vi "test-SetGetControlValue.vi"() -> (0 "errors":errorcluster[](array[cluster]))   [LabVIEW 2021]
uses:
  <vilib>/regexp/Match Regular Expression.xnode
panel:
  out "Variant":variant=variant(dbl 1.0)
  in  "Tab Control":enum32{"Page 1", "Page 2"}(tab)
  in  "Multiline\nwith\tTAB":string
  in  "NumericInPanel":dbl
  in  "Tab Control 2":enum32{"Page 1", "Page 2"}(tab)
  in  "StringInPanel":string
  in  "StringInPanel2":string
  in  "NumericInPanel2":dbl
  out "StringInd":string
  out "NumericInd":dbl
  in  "ClusterArray":cluster{"DBL":dbl, "U16":u16, "String":string}[](array[cluster])=[{"DBL"=2.0, "U16"=3, "String"="abc"}, {"DBL"=0.0, "U16"=0, "String"="aaa"}]
  in  "Cluster":T1={"DBL"=1.2, "U16"=3, "String"="bcd", "Ring U16"=3, "Ring EXT"=1.0, "Array"=[1.0, -1.0], "Boo/lean[2]"=FALSE} {"Ring EXT" items=["one", "three"]; "Ring U16" items=["one"=1, "three"=3]}
  in  "Array I32 2D":i32[][](array[numeric])=[[0, -1, 2], [3, 4, 5]]
  in  "Array I32":i32[](array[numeric])=[-1, 1, 2]
  in  "Enum":enum16{"zero", "one", "two"}(ring)
  in  "Ring 2":ext(ring)=3.3 items=["one", "three"]
  in  "Ring":u16(ring)=4 items=["one"=1, "three"=3]
  in  "Path":path
  in  "Combo Box 2":string(combo)="item1"
  in  "Combo Box":string(combo)="value1"
  in  "String":string="a\tb\nc\""
  in  "Radio Buttons":enum32{"Radio1", "Radio2"}(radio)
  in  "Boolean":bool
  in  "Color Box":u32(colorbox)
  in  "Scrollbar":dbl(c297)
  in  "Knob":dbl(knob) scale=0.0..10.0
  in  "Slide":dbl(slide) scale=0.0..10.0
  in  "Numeric U8":u8
  in  "Numeric CXT":cxt=10.0-0.30000000000000000001i
  in  "Numeric EXT":dbl=100.0
  out "Result":string="# Radio Buttons\nRadio Buttons=\"Radio2\"; Radio Buttons==\"Radio2\";\nRadio Buttons=0; Radio Buttons==\"Radio1\";"
  out "error":bool
  in  "CommandArray":T2(array[cluster])=[{"command"="# Numeric EXT 読み書きできるか\nNumeric EXT=3; Numeric EXT==3 # 一旦 3 にして\nNumeric EXT=0; Numeric EXT==0 # 0 に戻す", "result"="", "error"=FALSE}, {"command"="# Numeric EXT いろんな書き方\nNumeric EXT=1.0;Numeric EXT==1; # %f\nNumeric EXT=1E1;Numeric EXT==10; # %e\nNumeric EXT=\"1E2\";Numeric EXT==100; # 文字列でもOK", "result"="", "error"=FALSE}, {"command"="# 複素数\nNumeric CXT=1; Numeric CXT==\"1 +0 i\"\nNumeric CXT=-1; Numeric CXT==\"-1 +0 i\"\nNumeric CXT=\"0 +3.2 i\"; Numeric CXT==\"0 +3.2 i\"\nNumeric CXT=\"0 + i\"; Numeric CXT==\"0 +1 i\"\nNumeric CXT=\"0 - i\"; Numeric CXT==\"0 -1 i\"\nNumeric CXT=\"0 - 3.2 i\"; Numeric CXT==\"0 -3.2 i\"\nNumeric CXT=\"1e1 - 3e-1 i\"; Numeric CXT==\"10 -0.3 i\"", "result"="", "error"=FALSE}, {"command"="# Unsigned 8 bits\nNumeric U8=3; Numeric U8==3;\nNumeric U8=256; Numeric U8==255; # オーバーフローは飽和する\nNumeric U8=-2; Numeric U8==0; # アンダーフローも飽和する", "result"="", "error"=FALSE}, {"command"="# スライダー・Knob\nSlide=6; Slide==6; Slide=0; Slide==0; \nKnob=2; Knob==2; Knob=0; Knob==0", "result"="", "error"=FALSE}, {"command"="# Scrollbar\nScrollbar=10; Scrollbar==10;\nScrollbar=0.1; Scrollbar==0.1;\nScrollbar=0; Scrollbar==0;", "result"="", "error"=FALSE}, {"command"="# ColorBox\nColor Box=10000;Color Box==10000;\nColor Box=0;Color Box==0;", "result"="", "error"=FALSE}, {"command"="# Boolean\nBoolean=true; Boolean=false;\nBoolean=1; Boolean=0 # 数値でもいい", "result"="", "error"=FALSE}, {"command"="# Radio Buttons\nRadio Buttons=\"Radio2\"; Radio Buttons==\"Radio2\";\nRadio Buttons=0; Radio Buttons==\"Radio1\";", "result"="", "error"=FALSE}, {"command"="# String\nString=\"abc\"; String==\"abc\"; \nString=def; String==\"def\";  # これは許される\n# String=true; String==\"true\";  # これはエラーになる\n# String=0; String==\"0\";  # これらはエラーになる\nString=\"\"; String==\"\"; \nString=\"a\\tb\\nc\\\"\"; String==\"a\\tb\\nc\\\"\"; # エスケープシーケンス ", "result"="", "error"=FALSE}, {"command"="# Combo Box\nCombo Box=\"item1\"; Combo Box==\"item1\"; \nCombo Box=\"value1\"; Combo Box==\"value1\"; # 表示は item1 になる ", "result"="", "error"=FALSE}, {"command"="# Combo Box (Force Defined Value)\nCombo Box 2=\"item2\"; Combo Box 2==\"item2\"; \nCombo Box 2=\"\"; Combo Box 2==\"\"; \nCombo Box 2=\"value1\"; Combo Box 2==\"value1\"; # 表示は item1 になる\nCombo Box 2=\"undefined\"; Combo Box 2==\"undefined\"; # 代入する分には入れられる \nCombo Box 2=\"item1\"; Combo Box 2==\"item1\"; ", "result"="", "error"=FALSE}, {"command"="# Path\nPath=\"C:\\\\\"; Path==\"C:\\\\\"; \nPath=\"\"; Path==\"\"; ", "result"="", "error"=FALSE}, {"command"="# Ring\nRing=\"three\"; Ring==\"three\"; \nRing=\"one\"; Ring==\"one\"; \nRing=3; Ring==\"three\";  # 数値でも指定可能\nRing=0; Ring==\"<0>\"; # 範囲外の値も読み書きできる\nRing=\"<4>\"; Ring==\"<4>\"; # 文字列でもOK", "result"="", "error"=FALSE}, {"command"="# Ring メニュー（形は違うが機能は同じ？\nRing 2=\"three\"; Ring 2==\"three\"; \nRing 2=\"one\"; Ring 2==\"one\"; \nRing 2=3; Ring 2==\"three\";  # 数値でも指定可能\nRing 2=\"<3.2>\"; Ring 2==\"<3.2>\"\nRing 2=3.3; Ring 2==\"<3.3>\"", "result"="", "error"=FALSE}, {"command"="# Enum\nEnum=1; Enum==\"one\"\nEnum=\"two\"; Enum==\"two\"\nEnum=0; Enum==\"zero\"\nEnum=3; Enum==\"two\" # 範囲外の値は飽和する\nEnum=-1; Enum==\"zero\" # 範囲外の値は飽和する", "result"="", "error"=FALSE}, {"command"="# Array I32\nArray I32=[]; Array I32==[]\nArray I32=[0,1,2]; Array I32==[0,1,2]\nArray I32[0]=-1; Array I32==[-1,1,2]\n# Array I32[3]=-1; Array I32[-1]=-1 # Array index out of range エラーが出る", "result"="", "error"=FALSE}, {"command"="# Array I32 2D 多次元配列も可能\nArray I32 2D=[[0,0],[]]; Array I32 2D==[[0,0],[]]\nArray I32 2D=[[2,3],[0,1,2,3,4,5]];Array I32 2D==[[2,3],[0,1,2,3,4,5]]\nArray I32 2D[0,1]=-1;Array I32 2D==[[2,3],[0,-1,2,3,4,5]]\n# Array I32 2D[2,1]=-1; # Array index out of range.", "result"="", "error"=FALSE}, {"command"="# Cluster\nCluster={\"DBL\":0.1,\"U16\":3,\"String\":\"a\",\"Ring U16\":1, \"Ring EXT\":1,\"Array\":[]}\nCluster=={\"DBL\":0.1,\"U16\":3,\"String\":\"a\",\"Ring U16\":\"one\",\"Ring EXT\":\"one\",\"Array\":[]}\nCluster={0:0.2,3:\"three\"} # メンバー番号でもアクセスできる 一部のメンバーだけ指定してもいい\nCluster=={\"DBL\":0.2,\"U16\":3,\"String\":\"a\",\"Ring U16\":\"three\",\"Ring EXT\":\"one\",\"Array\":[]}\nCluster/DBL=1.2 # / でパスを指定して１つのメンバーだけにアクセスすることもできる\nCluster=={\"DBL\":1.2,\"U16\":3,\"String\":\"a\",\"Ring U16\":\"three\",\"Ring EXT\":\"one\",\"Array\":[]}\nCluster/DBL==1.2\nCluster/String=\"bcd\"\nCluster/String==\"bcd\"\nCluster/Array=[1,2]\nCluster/Array[1]=-1\nCluster/Array==[1,-1]", "result"="", "error"=FALSE}, {"command"="# ClusterArray\nClusterArray=[{DBL:2,U16:3,String:\"abc\"},{DBL:0,U16:-1,String:\"def\"}] # U16 に -1 は入らない\nClusterArray==[{\"DBL\":2,\"U16\":3,\"String\":\"abc\"},{\"DBL\":0,\"U16\":0,\"String\":\"def\"}]\nClusterArray[1]/DBL==0\nClusterArray[1]/String=\"aaa\"\nClusterArray[1]/String==\"aaa\"", "result"="", "error"=FALSE}, {"command"="# 表示器も扱える\nNumericInd=2; NumericInd==2\nNumericInd=0; NumericInd==0\nStringInd=\"aa\"; StringInd==\"aa\"\nStringInd=\"\"; StringInd==\"\"", "result"="", "error"=FALSE}, {"command"="# ページコントロールの各ページは平坦化される\nNumericInPanel=2; NumericInPanel==2; NumericInPanel=0; NumericInPanel==0\nNumericInPanel2=2; NumericInPanel2==2; NumericInPanel2=0; NumericInPanel2==0\nStringInPanel=\"aa\"; StringInPanel==\"aa\"; StringInPanel=\"\"; StringInPanel==\"\"\nStringInPanel2=\"aa\"; StringInPanel2==\"aa\"; StringInPanel2=\"\"; StringInPanel2==\"\"", "result"="", "error"=FALSE}, {"command"="# Sub Panel は一段下がる\nSub Panel/Numeric=1; Sub Panel/Numeric==1; Sub Panel/Numeric=0; Sub Panel/Numeric==0", "result"="", "error"=FALSE}, {"command"="# Variant 部分的なサポートしかない\n# 文字列、Boolean はOK。数値は部分的サポート。他は無理。\nVariant=\"abc\"; Variant==\"abc\"\nVariant=true; Variant==true\nVariant=false; Variant==false\n# 実数値も読み書きできるが書き込み時は常に EXT 型になる\nVariant=1.0; Variant==1", "result"="", "error"=FALSE}] caption="[テストスクリプト＆実行結果]\nテストスクリプトをここで一時的に変更して左上のボタンで再実行できるが\n内容は保存されないため必要ならダイアグラムのスクリプト欄を変更すること。"
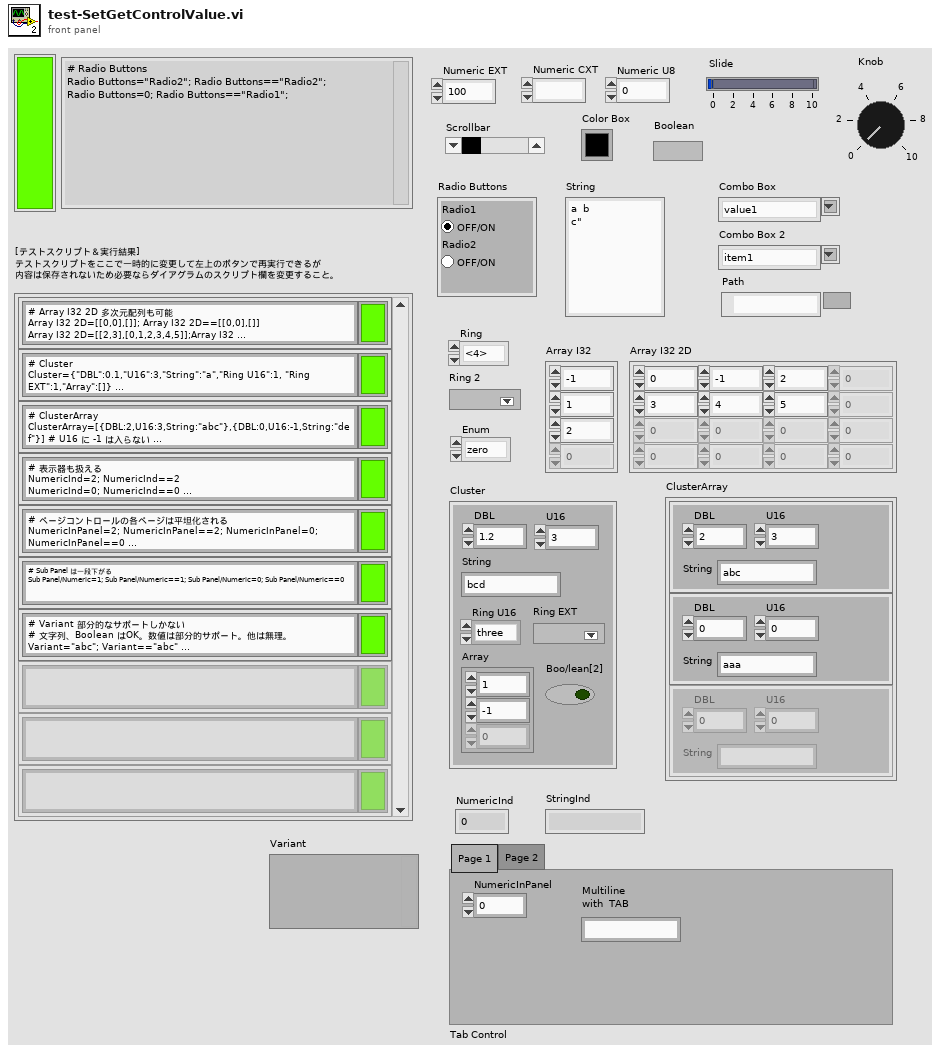
[diagram p1: front panel]
types:
  T1 = cluster{"DBL":dbl, "U16":u16, "String":string, "Ring U16":u16, "Ring EXT":ext, "Array":dbl[], "Boo/lean[2]":bool}
  T2 = cluster{"command":string, "result":string, "error":bool}[]
  T3 = cluster{"command":string, "result":string, "error":bool}
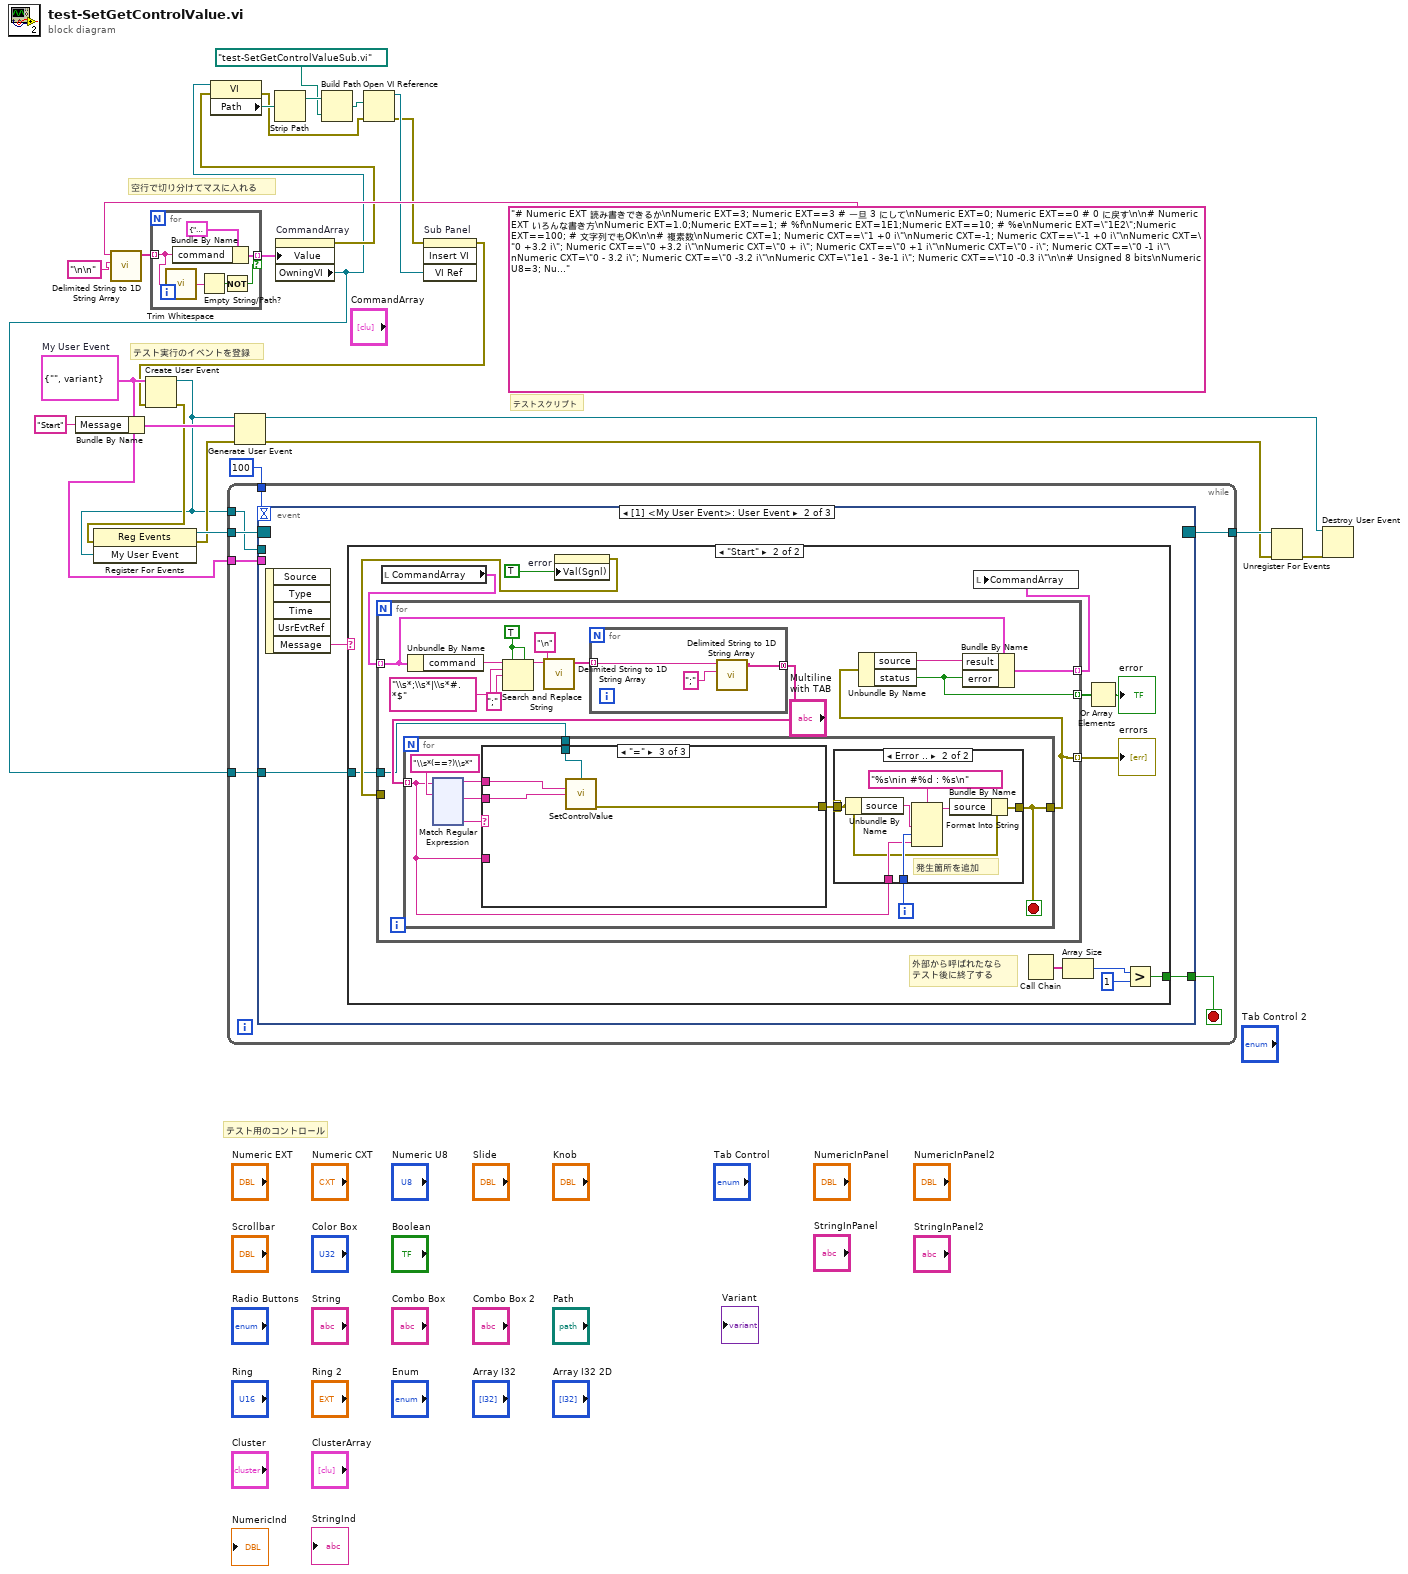
[diagram p0: block diagram]
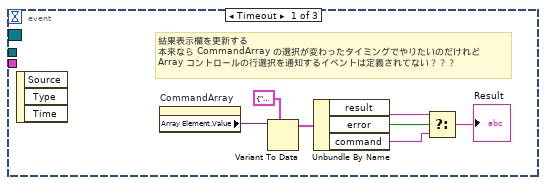
[diagram p2: hidden frame]
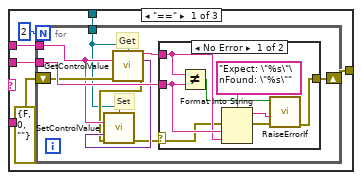
[diagram p5: hidden frame]
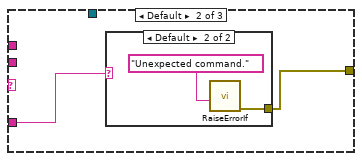
[diagram p7: hidden frame]
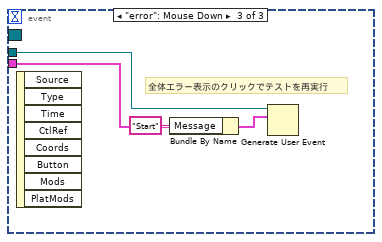
[diagram p9: hidden frame]
diagram:
  w16 = cluster{"Message":string, "Parameter":variant} {"Message"="", "Parameter"=variant}  # My User Event
  # "テスト用のコントロール"
  # "テスト実行のイベントを登録"
  # "空行で切り分けてマスに入れる"
  # "テストスクリプト"
  n1 = Bundle By Name(cluster=w16, "Message"="Start") -> (w19:cluster{"Message":string, "Parameter":variant})
  n2 = call <vilib>:"Delimited String to 1D String Array.vi"("delimiter"="\n\n", "delimited string"="# Numeric EXT 読み書きできるか\nNumeric EXT=3; Numeric EXT==3 # 一旦 3 にして\nNumeric EXT=0; Numeric EXT==0 # 0 に戻す\n\n# Numeric EXT いろんな書き方\nNumeric EXT=1.0;Numeric EXT==1; # %f\nNumeric EXT=1E1;Numeric EXT==10; # %e\nNumeric EXT=\"1E2\";Numeric EXT==100; # 文字列でもOK\n\n# 複素数\nNumeric CXT=1; Numeric CXT==\"1 +0 i\"\nNumeric CXT=-1; Numeric CXT==\"-1 +0 i\"\nNumeric CXT=\"0 +3.2 i\"; Numeric CXT==\"0 +3.2 i\"\nNumeric CXT=\"0 + i\"; Numeric CXT==\"0 +1 i\"\nNumeric CXT=\"0 - i\"; Numeric CXT==\"0 -1 i\"\nNumeric CXT=\"0 - 3.2 i\"; Numeric CXT==\"0 -3.2 i\"\nNumeric CXT=\"1e1 - 3e-1 i\"; Numeric CXT==\"10 -0.3 i\"\n\n# Unsigned 8 bits\nNumeric U8=3; Numeric U8==3;\nNumeric U8=256; Numeric U8==255; # オーバーフローは飽和する\nNumeric U8=-2; Numeric U8==0; # アンダーフローも飽和する\n\n# スライダー・Knob\nSlide=6; Slide==6; Slide=0; Slide==0; \nKnob=2; Knob==2; Knob=0; Knob==0\n\n# Scrollbar\nScrollbar=10; Scrollbar==10;\nScrollbar=0.1; Scrollbar==0.1;\nScrollbar=0; Scrollbar==0;\n\n# ColorBox\nColor Box=10000;Color Box==10000;\nColor Box=0;Color Box==0;\n\n# Boolean\nBoolean=true; Boolean=false;\nBoolean=1; Boolean=0 # 数値でもいい\n\n# Radio Buttons\nRadio Buttons=\"Radio2\"; Radio Buttons==\"Radio2\";\nRadio Buttons=0; Radio Buttons==\"Radio1\";\n\n# String\nString=\"abc\"; String==\"abc\"; \nString=def; String==\"def\";  # これは許される\n# String=true; String==\"true\";  # これはエラーになる\n# String=0; String==\"0\";  # これらはエラーになる\nString=\"\"; String==\"\"; \nString=\"a\\tb\\nc\\\"\"; String==\"a\\tb\\nc\\\"\"; # エスケープシーケンス \n\n# Combo Box\nCombo Box=\"item1\"; Combo Box==\"item1\"; \nCombo Box=\"value1\"; Combo Box==\"value1\"; # 表示は item1 になる \n\n# Combo Box (Force Defined Value)\nCombo Box 2=\"item2\"; Combo Box 2==\"item2\"; \nCombo Box 2=\"\"; Combo Box 2==\"\"; \nCombo Box 2=\"value1\"; Combo Box 2==\"value1\"; # 表示は item1 になる\nCombo Box 2=\"undefined\"; Combo Box 2==\"undefined\"; # 代入する分には入れられる \nCombo Box 2=\"item1\"; Combo Box 2==\"item1\"; \n\n# Path\nPath=\"C:\\\\\"; Path==\"C:\\\\\"; \nPath=\"\"; Path==\"\"; \n\n# Ring\nRing=\"three\"; Ring==\"three\"; \nRing=\"one\"; Ring==\"one\"; \nRing=3; Ring==\"three\";  # 数値でも指定可能\nRing=0; Ring==\"<0>\"; # 範囲外の値も読み書きできる\nRing=\"<4>\"; Ring==\"<4>\"; # 文字列でもOK\n\n# Ring メニュー（形は違うが機能は同じ？\nRing 2=\"three\"; Ring 2==\"three\"; \nRing 2=\"one\"; Ring 2==\"one\"; \nRing 2=3; Ring 2==\"three\";  # 数値でも指定可能\nRing 2=\"<3.2>\"; Ring 2==\"<3.2>\"\nRing 2=3.3; Ring 2==\"<3.3>\"\n\n# Enum\nEnum=1; Enum==\"one\"\nEnum=\"two\"; Enum==\"two\"\nEnum=0; Enum==\"zero\"\nEnum=3; Enum==\"two\" # 範囲外の値は飽和する\nEnum=-1; Enum==\"zero\" # 範囲外の値は飽和する\n\n# Array I32\nArray I32=[]; Array I32==[]\nArray I32=[0,1,2]; Array I32==[0,1,2]\nArray I32[0]=-1; Array I32==[-1,1,2]\n# Array I32[3]=-1; Array I32[-1]=-1 # Array index out of range エラーが出る\n\n# Array I32 2D 多次元配列も可能\nArray I32 2D=[[0,0],[]]; Array I32 2D==[[0,0],[]]\nArray I32 2D=[[2,3],[0,1,2,3,4,5]];Array I32 2D==[[2,3],[0,1,2,3,4,5]]\nArray I32 2D[0,1]=-1;Array I32 2D==[[2,3],[0,-1,2,3,4,5]]\n# Array I32 2D[2,1]=-1; # Array index out of range.\n\n# Cluster\nCluster={\"DBL\":0.1,\"U16\":3,\"String\":\"a\",\"Ring U16\":1, \"Ring EXT\":1,\"Array\":[],\"Boo/lean[2]\":false}\nCluster=={\"DBL\":0.1,\"U16\":3,\"String\":\"a\",\"Ring U16\":\"one\",\"Ring EXT\":\"one\",\"Array\":[],\"Boo/lean[2]\":false}\nCluster={0:0.2,3:\"three\",\"Boo/lean[2]\":true} # メンバー番号でもアクセスできる 一部のメンバーだけ指定してもいい\nCluster=={\"DBL\":0.2,\"U16\":3,\"String\":\"a\",\"Ring U16\":\"three\",\"Ring EXT\":\"one\",\"Array\":[],\"Boo/lean[2]\":true}\nCluster/DBL=1.2 # / でパスを指定して１つのメンバーだけにアクセスすることもできる\nCluster=={\"DBL\":1.2,\"U16\":3,\"String\":\"a\",\"Ring U16\":\"three\",\"Ring EXT\":\"one\",\"Array\":[],\"Boo/lean[2]\":true}\nCluster/DBL==1.2\nCluster/String=\"bcd\"\nCluster/String==\"bcd\"\nCluster/Array=[1,2]\nCluster/Array[1]=-1\nCluster/Array==[1,-1]\nCluster/Boo\\/lean\\[2]=false # / [ を含むコントロール名をパスで指定する際には \\ でエスケープする\nCluster/Boo\\/lean\\[2]==false\n\n# ClusterArray\nClusterArray=[{DBL:2,U16:3,String:\"abc\"},{DBL:0,U16:-1,String:\"def\"}] # U16 に -1 は入らない\nClusterArray==[{\"DBL\":2,\"U16\":3,\"String\":\"abc\"},{\"DBL\":0,\"U16\":0,\"String\":\"def\"}]\nClusterArray[1]/DBL==0\nClusterArray[1]/String=\"aaa\"\nClusterArray[1]/String==\"aaa\"\n\n# 表示器も扱える\nNumericInd=2; NumericInd==2\nNumericInd=0; NumericInd==0\nStringInd=\"aa\"; StringInd==\"aa\"\nStringInd=\"\"; StringInd==\"\"\n\n# ページコントロールの各ページは平坦化される\nNumericInPanel=2; NumericInPanel==2; NumericInPanel=0; NumericInPanel==0\nNumericInPanel2=2; NumericInPanel2==2; NumericInPanel2=0; NumericInPanel2==0\nStringInPanel=\"aa\"; StringInPanel==\"aa\"; StringInPanel=\"\"; StringInPanel==\"\"\nStringInPanel2=\"aa\"; StringInPanel2==\"aa\"; StringInPanel2=\"\"; StringInPanel2==\"\"\n\n# Sub Panel は一段下がる\nSub Panel/Numeric=1; Sub Panel/Numeric==1\nSub Panel/Numeric=0; Sub Panel/Numeric==0\n\n# Variant 部分的なサポートしかない\n# 文字列、Boolean はOK。数値は部分的サポート。他は無理。\nVariant=\"abc\"; Variant==\"abc\"\nVariant=true; Variant==true\nVariant=false; Variant==false\n# 実数値も読み書きできるが書き込み時は常に EXT 型になる\nVariant=1.0; Variant==1\n\n# Tab Control のページを選択できる(数値かページ名)\nTab Control=1; Tab Control==\"Page 2\"\nTab Control=0; Tab Control==\"Page 1\"\nTab Control=\"Page 2\"; Tab Control==\"Page 2\"\n\n# 名前のエスケープ\nMultiline\\nwith\\tTAB=\"\"; Multiline\\nwith\\tTAB==\"\"\nMultiline\\nwith\\tTAB=\"Hello!\"; Multiline\\nwith\\tTAB==\"Hello!\"\n" ("Script")) -> ("string array"=w13:string[])  [unwired: 9 in]
  n3 = for {
    tunnel: w13 -> [w27] mode=indexing
    tunnel: [w32] -> w12 mode=indexing if=w29
    n4 = call <vilib>:"Trim Whitespace.vi"("string"=w27) -> ("trimmed string"=w28:string)  [unwired: 1 in]
    n5 = Bundle By Name(cluster=T3 {"command"="", "result"="", "error"=FALSE} ("Cluster"), "command"=w27) -> (w32:T3)
    n6 = Empty String/Path?(string/path=w28) -> (empty?=w30:bool)
    n7 = Not(x=w30) -> (.not. x?=w29:bool)
  }
  n8 = property on="CommandArray" class="Arr (strict)"("Value"=w12) -> (error out=w4:errorcluster, "OwningVI"=w1:refnum<vi>)  [unwired: 2 in, 1 out]
  n9 = property class="VI"(reference=w1, error in=w4) -> (error out=w3:errorcluster, "Path"=w9:path)  [unwired: 1 out]
  n10 = Strip Path(path=w9) -> (stripped path=w8:path)  [unwired: 1 out]
  n11 = Build Path(base path=w8, name or relative path=path "test-SetGetControlValueSub.vi") -> (appended path=w6:path)
  n12 = Open VI Reference(vi path=w6, error in (no error)=w3) -> (vi reference=w5:refnum<vi>, error out=w2:errorcluster)  [unwired: 4 in]
  n13 = invoke on="Sub Panel" class="SubPnl" method="Insert VI"(error in=w2, "VI Ref"=w5) -> (error out=w10:errorcluster)  [unwired: 2 in, 3 out]
  n14 = Create User Event(user event datatype=w16, error in=w10) -> (user event=w17:refnum<user-event>, error out=w18:errorcluster)
  n15 = register-events(error in=w18, w17) -> (reference out=w26:refnum<event-registration>, error out=w24:errorcluster)  [unwired: 1 in]
  n16 = while {
    tunnel: w26 -> [w39]
    tunnel: [w38] -> w25
    tunnel: w17 -> [w37]
    tunnel: w16 -> [w36]
    tunnel: 100 -> [w35]
    tunnel: w1 -> [w33]
    stop <- w34 stop-if-true
    n17 = event shown="[1] <My User Event>: User Event" {
      selector: w39 -> [_ _ _]
      dyn-events: [_ _ _] -> w38
      timeout: w35 -> [_ _ _]
      tunnel: w37 -> [_ _ w251]
      tunnel: w36 -> [_ _ w249]
      tunnel: [_ w48 _] -> w34
      tunnel: w33 -> [_ w47 _]
      event Timeout {
        # "結果表示欄を更新する\n本来なら CommandArray の選択が変わったタイミングでやりたいのだけれど\nArray コントロールの行選択を通知するイベントは定義されてない？？？"
        n18 = event-data() -> ()  [unwired: 1 in, 3 out]
        n19 = property on="CommandArray" class="Arr (strict)"() -> ("Array Element.Value"=w46:variant)  [unwired: 2 in, 2 out]
        n20 = Variant To Data(type=T3 {"command"="", "result"="", "error"=FALSE} ("Cluster"), Variant=w46) -> (data=w44:T3)  [unwired: 1 in, 1 out]
        n21 = Unbundle By Name(w44) -> ("result"=w42:string, "error"=w43:bool, "command"=w41:string)
        n22 = Select(t=w42, s=w43, f=w41) -> (s? t:f=→"Result":string)
      }
      event User Event {
        n23 = event-data() -> ("Message"=w49:string)  [unwired: 1 in, 4 out]
        n24 = case shown="\"Start\"" w49 {
          tunnel: [_ w53] -> w48
          tunnel: w47 -> [_ w50]
          frame Default {
          }
          frame "Start" {
            # "外部から呼ばれたなら\nテスト後に終了する"
            n25 = local read "CommandArray"() -> (w61:T2)
            n26 = property on="error" class="Bool (strict)"("Val(Sgnl)"=TRUE ("Value (Signaling)")) -> (error out=w51:errorcluster)  [unwired: 2 in, 1 out]
            n27 = for {
              tunnel: w61 -> [w69] mode=indexing
              tunnel: [w67] -> w60 mode=indexing
              tunnel: [w66] -> w59 mode=indexing
              tunnel: [w63] -> w57 mode=indexing
              tunnel: w51 -> [_]
              tunnel: w50 -> [w62]
              w64 = TRUE ("replace all? (F)")
              n28 = Unbundle By Name(w69) -> ("command"=w72:string)
              n29 = Search and Replace String(replace all?=w64, multiline?=w64, input string=w72, search string="\\s*;\\s*|\\s*#.*$", replace string=";" ("replace string (\"\")")) -> (result string=w65:string)  [unwired: 3 in, 3 out]
              n30 = call <vilib>:"Delimited String to 1D String Array.vi"("delimiter"="\n", "delimited string"=w65) -> ("string array"=w74:string[])  [unwired: 9 in]
              n31 = for {
                tunnel: w74 -> [w245] mode=indexing
                tunnel: [w247] -> w70 mode=concatenating
                n32 = call <vilib>:"Delimited String to 1D String Array.vi"("delimiter"=";", "delimited string"=w245) -> ("string array"=w247:string[])  [unwired: 9 in]
              }
              n33 = for {
                tunnel: w70 -> [w77] mode=indexing
                tunnel: [w79] -> w63
                tunnel: w62 -> [w76]
                i -> [w80]
                stop <- w79 stop-if-true
                n34 = xnode "Match Regular Expression"("input string"=w77, "regular expression"="\\s*(==?)\\s*") -> ("before match"=w83:string, "after match"=w82:string, "submatch 1"=w78:string)  [unwired: 4 in, 3 out]
                n35 = case shown="\"=\"" w78 {
                  tunnel: w83 -> [w99 _ w125]
                  tunnel: w82 -> [w98 _ w124]
                  tunnel: [w97 w119 w123] -> w81
                  tunnel: w77 -> [_ w118 _]
                  tunnel: w76 -> [w94 _ w122]
                  frame "==" {
                    n36 = for {
                      N: 2 -> [_]
                      tunnel: w99 -> [w104]
                      tunnel: w98 -> [w107]
                      shift-right: [w106] -> w97
                      shift-left: errorcluster {"status"=FALSE, "code"=0, "source"=""} ("error IO") -> [w105]
                      tunnel: w94 -> [w100]
                      # "Set"
                      # "Get"
                      n37 = call "GetControlValue.vi"("vi ref"=w100, "ctrl"=w104, "error in (no error)"=w105) -> ("String out"=w108:string, "value"=w103:variant, "error out"=w102:errorcluster)  [unwired: 10 in]
                      n38 = call "SetControlValue.vi"("vi ref"=w100, "ctrl"=w104, "Value"=w103, "error in (no error)"=w102) -> ("error out"=w101:errorcluster)  [unwired: 11 in]
                      n39 = case shown="No Error" w101 {
                        selector: w101 -> [w110 w117]
                        tunnel: w108 -> [w114 _]
                        tunnel: w107 -> [w115 _]
                        tunnel: [w111 w117] -> w106
                        frame No Error {
                          n40 = Not Equal?(x=w114, y=w115) -> (x != y?=w113:bool)
                          n41 = Format Into String(format string="Expect: \"%s\"\nFound: \"%s\"", error in=w110, w115, w114) -> (resulting string=w112:string, error out=w109:errorcluster)  [unwired: 1 in]
                          n42 = call "RaiseErrorIf.vi"("error in (no error)"=w109, "error message"=w112, "error? (true)"=w113) -> ("error out"=w111:errorcluster)  [unwired: 8 in]
                        }
                        frame Error {
                        }
                      }
                    }
                  }
                  frame Default {
                    n43 = case shown="Default" w118 {
                      tunnel: [_ w121] -> w119
                      frame "" {
                      }
                      frame Default {
                        n44 = call "RaiseErrorIf.vi"("error message"="Unexpected command." ("format string")) -> ("error out"=w121:errorcluster)  [unwired: 10 in]
                      }
                    }
                  }
                  frame "=" {
                    n45 = call "SetControlValue.vi"("vi ref"=w122, "ctrl"=w125, "Value (JSON)"=w124) -> ("error out"=w123:errorcluster)  [unwired: 12 in]
                  }
                }
                n46 = case shown="Error .." w81 {
                  selector: w81 -> [w85 w87]
                  tunnel: w81 -> [_ w93]
                  tunnel: w80 -> [_ w90]
                  tunnel: w77 -> [_ w89]
                  tunnel: [w85 w86] -> w79
                  frame No Error {
                  }
                  frame Error {
                    # "発生箇所を追加"
                    n47 = Unbundle By Name(w93) -> ("source"=w91:string)
                    n48 = Format Into String(format string="%s\nin #%d : %s\n", w91, w90, w89) -> (resulting string=w88:string)  [unwired: 2 in, 1 out]
                    n49 = Bundle By Name(cluster=w87, "source"=w88) -> (w86:errorcluster)
                  }
                }
              }
              n50 = Unbundle By Name(w63) -> ("source"=w68:string, "status"=w66:bool)
              n51 = Bundle By Name(cluster=w69, "result"=w68, "error"=w66) -> (w67:T3)
            }
            "errors" <- w57
            n52 = local write "CommandArray"(w60) -> ()
            n53 = Call Chain() -> (call chain=w55:string[])
            n54 = Array Size(array=w55) -> (size(s)=w56:i32)
            n55 = Or Array Elements(Boolean array=w59) -> (logical OR=→"error":bool)
            n56 = Greater?(x=w56, y=1) -> (0:w53:bool)
          }
        }
      }
      event "error": Mouse Down {
        # "全体エラー表示のクリックでテストを再実行"
        n57 = event-data() -> ()  [unwired: 1 in, 8 out]
        n58 = Bundle By Name(cluster=w249, "Message"="Start") -> (w248:cluster{"Message":string, "Parameter":variant})
        n59 = Generate User Event(user event=w251, event data cluster=w248) -> ()  [unwired: 2 in, 2 out]
      }
    }
  }
  n60 = Generate User Event(user event=w17, event data cluster=w19, error in=w24) -> (user event out=w23:refnum<user-event>, error out=w22:errorcluster)  [unwired: 1 in]
  n61 = Unregister For Events(event registration refnum=w25, error in=w22) -> (error out=w21:errorcluster)
  n62 = Destroy User Event(user event=w23, error in=w21) -> ()  [unwired: 1 out]
